vi "read 4 bytes.vi"() -> ()   [LabVIEW 2019]
panel:
  out "Z  axis RAW values":i16
  out "Y  axis RAW values":i16
  out "X axis RAW values":i16
  out "high z axis":u8 format="%x"
  out "low z axis":u8 format="%x"
  out "high y axis":u8 format="%x"
  out "low y axis":u8 format="%x"
  out "High X axis":u8 format="%x"
  out "low X axis  2":u8 format="%x"
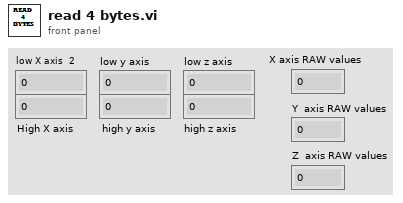
[diagram p1: front panel]
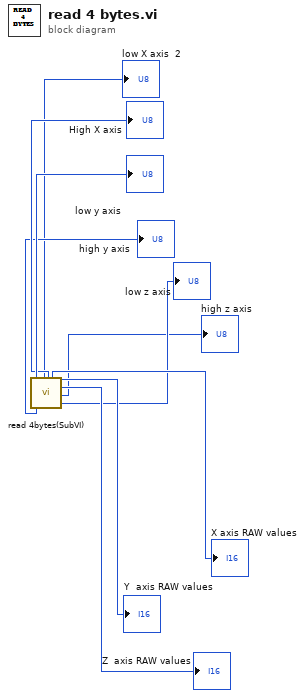
[diagram p0: block diagram]
diagram:
  n1 = call "read 4bytes(SubVI).vi"() -> ("low y axis"=→"low y axis":u8, "high y axis"=→"high y axis":u8, "low X axis  2"=→"low X axis  2":u8, "High X axis"=→"High X axis":u8, "Numeric 3"=→"X axis RAW values":i16, "Numeric 2"=→"Y  axis RAW values":i16, "Numeric"=→"Z  axis RAW values":i16, "high z axis"=→"high z axis":u8, "low z axis"=→"low z axis":u8)  [unwired: 7 in, 12 out]
